vi "numCmd_Send_Array.vi"(7 "Command Name":string, 11 "Values":dbl[](array[numeric])) -> (0 "error out":errorcluster)   [LabVIEW 2019, in "Trajectory_Library.lvlib"]
uses:
  Trajectory_Library.lvlib
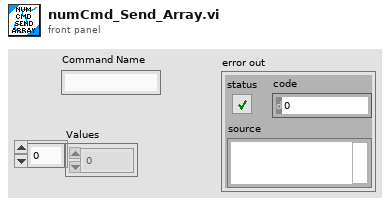
[diagram p1: front panel]
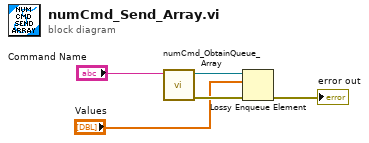
[diagram p0: block diagram]
diagram:
  n1 = call "numCmd_ObtainQueue_Array.vi"("Command Name"="Command Name") -> ("error out"=w4:errorcluster, "queue out"=w5:refnum<queue>)  [unwired: 9 in]
  n2 = Lossy Enqueue Element(queue=w5, element="Values", error in (no error)=w4) -> (error out=→"error out":errorcluster)  [unwired: 3 out]
